vi "IFD Image Input.vi"(8 "error in (no error)":errorcluster, 9 "Data type":T1, 10 "size(s)":i32[](array[numeric]), 11 "IFD in":refnum<class "IFD.lvclass">) -> (0 "error out":errorcluster, 3 "IFD out":refnum<class "IFD.lvclass">)   [LabVIEW 2016, in "IFD.lvclass"]
uses:
  IFD.lvclass
  Img Data Type.ctl
  IFD.lvclass/IFD.ctl
  Tag/IFD_Tag.lvclass/IFD_Tag.ctl
  Tag/IFD_Tag.lvclass
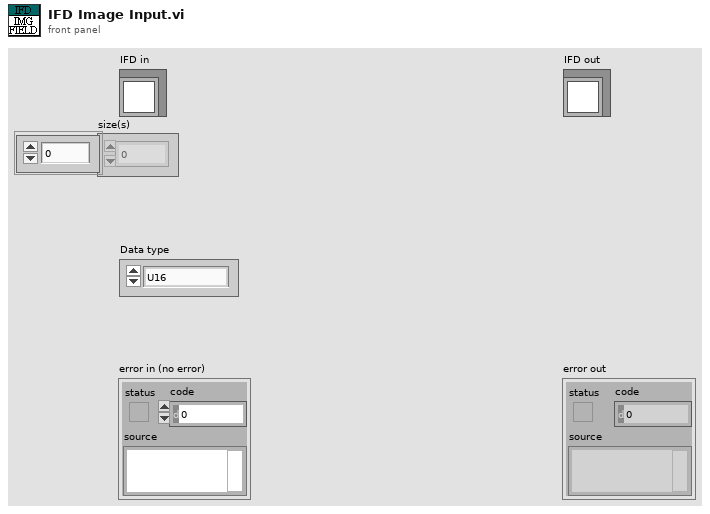
[diagram p1: front panel]
types:
  T1 = typedef "Img Data Type.ctl" = enum16{"U16", "RGB", "SGL"}
  T2 = enum16{"Undefined(DO NOT USE)", "U8", "ASCII", "U16", "U32", "RATIONAL", "I8", "Undefined 8 bit", "I16", "I32", "SRATIONAL", "SGL", "DBL"}
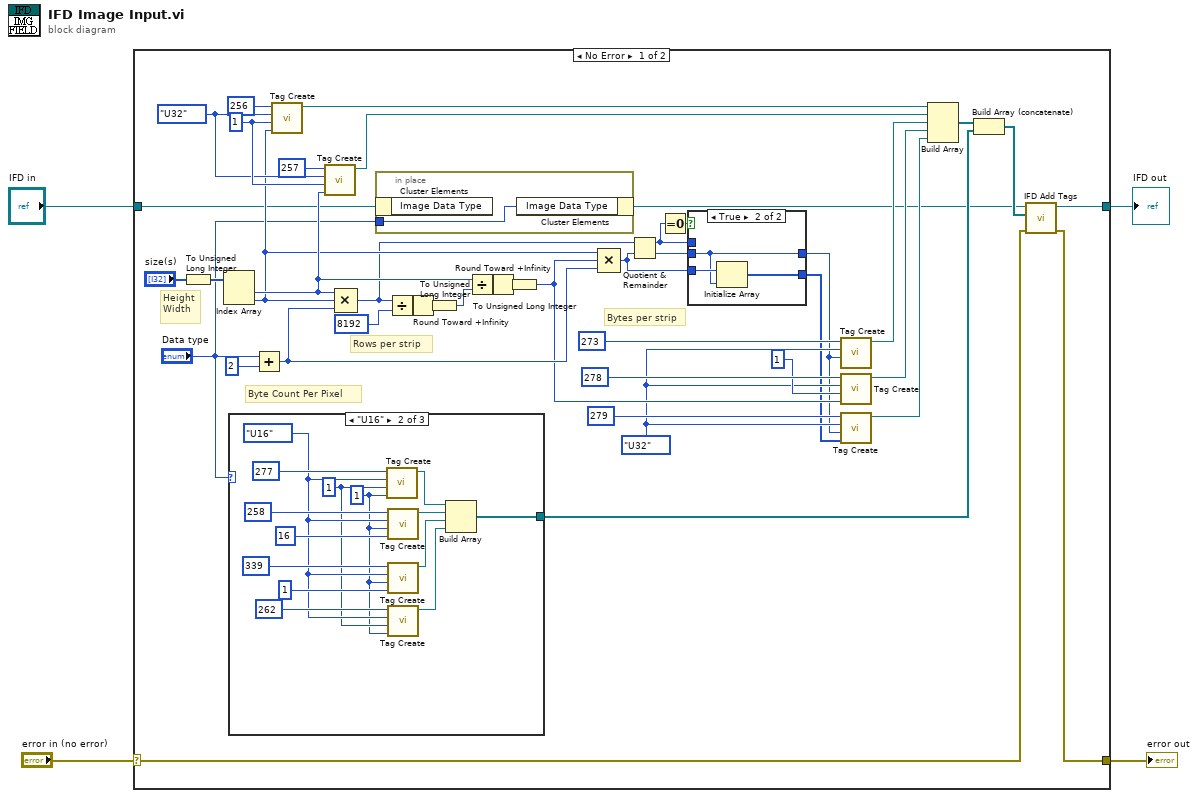
[diagram p0: block diagram]
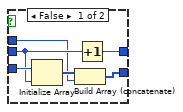
[diagram p2: hidden frame]
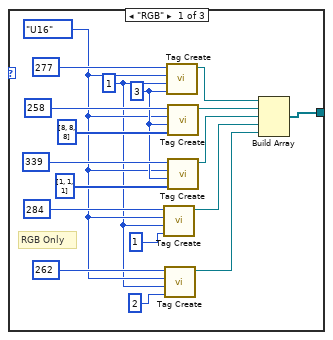
[diagram p3: hidden frame]
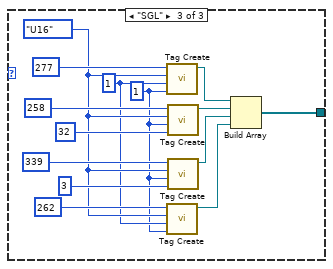
[diagram p4: hidden frame]
diagram:
  n1 = case shown="No Error" "error in (no error)" {
    selector: "error in (no error)" -> [w38 w105]
    tunnel: [w37 w105] -> w3
    tunnel: [w47 w104] -> w1
    tunnel: "IFD in" -> [w7 w104]
    frame No Error {
      w16 = T2."U32" ("Data Type")
      w42 = u32 1 ("Data Count")
      w41 = T2."U32" ("Data Type")
      # "Bytes per strip"
      # "Rows per strip"
      # "Byte Count Per Pixel"
      # "Height\nWidth"
      n2 = To Unsigned Long Integer(number="size(s)") -> (unsigned 32bit integer=w34:u32[])
      n3 = Index Array(array=w34) -> (element #1=w31:u32, element #2=w27:u32)  [unwired: 2 in]
      n4 = case shown="\"U16\"" "Data type" {
        tunnel: [w63 w81 w95] -> w8
        frame "RGB" {
          w70 = u16 3
          w60 = u32 1 ("Data Count")
          w61 = T2."U16" ("Data Type")
          # "RGB Only"
          n5 = call "Tag Create.vi"("Data"=u16 1, "Data Count"=w60, "Data Type"=w61, "Tag ID"=u16 284) -> ("IFD_Tag out"=w64:refnum<class "IFD_Tag.lvclass">)  [unwired: 7 in]
          n6 = call "Tag Create.vi"("Data"=u16 2, "Data Count"=w60, "Data Type"=w61, "Tag ID"=u16 262) -> ("IFD_Tag out"=w58:refnum<class "IFD_Tag.lvclass">)  [unwired: 7 in]
          n7 = call "Tag Create.vi"("Data"=w70, "Data Count"=w60, "Data Type"=w61, "Tag ID"=u16 277) -> ("IFD_Tag out"=w67:refnum<class "IFD_Tag.lvclass">)  [unwired: 7 in]
          n8 = call "Tag Create.vi"("Data"=u16[] [8, 8, 8], "Data Count"=w70, "Data Type"=w61, "Tag ID"=u16 258) -> ("IFD_Tag out"=w66:refnum<class "IFD_Tag.lvclass">)  [unwired: 7 in]
          n9 = call "Tag Create.vi"("Data"=u16[] [1, 1, 1], "Data Count"=w70, "Data Type"=w61, "Tag ID"=u16 339) -> ("IFD_Tag out"=w65:refnum<class "IFD_Tag.lvclass">)  [unwired: 7 in]
          n10 = Build Array(w67, w66, w65, w64, w58) -> (w63:refnum<class "IFD_Tag.lvclass">[])
        }
        frame "U16" {
          w76 = u16 1
          w77 = u32 1 ("Data Count")
          w78 = T2."U16" ("Data Type")
          n11 = call "Tag Create.vi"("Data"=w76, "Data Count"=w77, "Data Type"=w78, "Tag ID"=u16 277) -> ("IFD_Tag out"=w84:refnum<class "IFD_Tag.lvclass">)  [unwired: 7 in]
          n12 = call "Tag Create.vi"("Data"=u16 16, "Data Count"=w76, "Data Type"=w78, "Tag ID"=u16 258) -> ("IFD_Tag out"=w83:refnum<class "IFD_Tag.lvclass">)  [unwired: 7 in]
          n13 = call "Tag Create.vi"("Data"=u16 1, "Data Count"=w76, "Data Type"=w78, "Tag ID"=u16 339) -> ("IFD_Tag out"=w82:refnum<class "IFD_Tag.lvclass">)  [unwired: 7 in]
          n14 = call "Tag Create.vi"("Data"=w76, "Data Count"=w77, "Data Type"=w78, "Tag ID"=u16 262) -> ("IFD_Tag out"=w79:refnum<class "IFD_Tag.lvclass">)  [unwired: 7 in]
          n15 = Build Array(w84, w83, w82, w79) -> (w81:refnum<class "IFD_Tag.lvclass">[])
        }
        frame "SGL" {
          w90 = u16 1
          w91 = u32 1 ("Data Count")
          w92 = T2."U16" ("Data Type")
          n16 = call "Tag Create.vi"("Data"=w90, "Data Count"=w91, "Data Type"=w92, "Tag ID"=u16 277) -> ("IFD_Tag out"=w98:refnum<class "IFD_Tag.lvclass">)  [unwired: 7 in]
          n17 = call "Tag Create.vi"("Data"=w90, "Data Count"=w91, "Data Type"=w92, "Tag ID"=u16 262) -> ("IFD_Tag out"=w93:refnum<class "IFD_Tag.lvclass">)  [unwired: 7 in]
          n18 = call "Tag Create.vi"("Data"=u16 32, "Data Count"=w90, "Data Type"=w92, "Tag ID"=u16 258) -> ("IFD_Tag out"=w97:refnum<class "IFD_Tag.lvclass">)  [unwired: 7 in]
          n19 = call "Tag Create.vi"("Data"=u16 3, "Data Count"=w90, "Data Type"=w92, "Tag ID"=u16 339) -> ("IFD_Tag out"=w96:refnum<class "IFD_Tag.lvclass">)  [unwired: 7 in]
          n20 = Build Array(w98, w97, w96, w93) -> (w95:refnum<class "IFD_Tag.lvclass">[])
        }
      }
      n21 = Add(x="Data type", y=u32 2) -> (x+y=w26:u32)
      n22 = call "Tag Create.vi"("Data"=w27, "Data Count"=w42, "Data Type"=w41, "Tag ID"=u16 256) -> ("IFD_Tag out"=w44:refnum<class "IFD_Tag.lvclass">)  [unwired: 7 in]
      n23 = call "Tag Create.vi"("Data"=w31, "Data Count"=w42, "Data Type"=w41, "Tag ID"=u16 257) -> ("IFD_Tag out"=w43:refnum<class "IFD_Tag.lvclass">)  [unwired: 7 in]
      n24 = Compound Arithmetic op=MULTIPLY(w31, w27, w26) -> (w24:u32)
      n25 = in-place {
        in-place-border: "Data type" -> [w48]
        n26 = in-place-cluster #1(w7) -> ()  [unwired: 1 out]
        n27 = in-place-cluster #1("Image Data Type"=w48) -> (w6:refnum<class "IFD.lvclass">)
      }
      n28 = Divide(x=w24, y=u32 8192) -> (x/y=w32:dbl)
      n29 = Round Toward +Infinity(x=w32) -> (ceil(x): smallest int >= x=w29:dbl)
      n30 = To Unsigned Long Integer(number=w29) -> (unsigned 32bit integer=w25:u32)
      n31 = Divide(x=w31, y=w25) -> (x/y=w30:dbl)
      n32 = Round Toward +Infinity(x=w30) -> (ceil(x): smallest int >= x=w28:dbl)
      n33 = To Unsigned Long Integer(number=w28) -> (unsigned 32bit integer=w19:u32)
      n34 = Compound Arithmetic op=MULTIPLY(w27, w19, w26) -> (w10:u32)
      n35 = Quotient & Remainder(x=w24, y=w10) -> (x-y*floor(x/y)=w12:u32, floor(x/y)=w13:u32)
      n36 = Equal To 0?(x=w12) -> (x = 0?=w14:bool)
      n37 = case shown="True" w14 {
        tunnel: w13 -> [w52 w56]
        tunnel: w12 -> [w49 _]
        tunnel: [w54 w56] -> w11
        tunnel: w10 -> [w53 w57]
        tunnel: [w50 w55] -> w9
        frame False {
          n38 = Initialize Array(w53, w52) -> (w51:u32[])
          n39 = Build Array (concatenate)(w51, w49) -> (w50:u32[])
          n40 = Increment(x=w52) -> (x+1=w54:u32)
        }
        frame True {
          n41 = Initialize Array(w57, w56) -> (w55:u32[])
        }
      }
      n42 = call "Tag Create.vi"("Data Count"=w11, "Data Type"=w16, "Tag ID"=u16 273) -> ("IFD_Tag out"=w22:refnum<class "IFD_Tag.lvclass">)  [unwired: 8 in]
      n43 = call "Tag Create.vi"("Data"=w19, "Data Count"=u32 1, "Data Type"=w16, "Tag ID"=u16 278) -> ("IFD_Tag out"=w18:refnum<class "IFD_Tag.lvclass">)  [unwired: 7 in]
      n44 = call "Tag Create.vi"("Data"=w9, "Data Count"=w11, "Data Type"=w16, "Tag ID"=u16 279) -> ("IFD_Tag out"=w15:refnum<class "IFD_Tag.lvclass">)  [unwired: 7 in]
      n45 = Build Array(w44, w43, w22, w18, w15) -> (w40:refnum<class "IFD_Tag.lvclass">[])
      n46 = Build Array (concatenate)(w40, w8) -> (w39:refnum<class "IFD_Tag.lvclass">[])
      n47 = call "IFD Add Tags.vi"("error in (no error)"=w38, "Tag(s)"=w39, "IFD in"=w6) -> ("error out"=w37:errorcluster, "IFD out"=w47:refnum<class "IFD.lvclass">)  [unwired: 7 in]
    }
    frame Error {
    }
  }
  "error out" <- w3
  "IFD out" <- w1
